vi "STM32.cmd.vi"(8 "Error In":errorcluster caption="错误输入", 10 "命令":string, 11 "VISA资源输入":refnum<visa-resource-name>) -> (0 "Error Out":errorcluster caption="错误输出", 1 "附加数据":string, 2 "返回":string, 3 "返回长度":u32)   [LabVIEW 2012, in "Lib_UEL.ATE.lvlib" / "STM32-CoreBD.lvlib"]
uses:
  STM32-CoreBD.lvlib
  <vilib>/Instr/_visa.llb/VISA Open Access Mode.ctl
panel:
  out "返回数":u32
  out "附加读取长度":u32
  out "读取缓冲区":string
  out "发送长度":u32
  out "错误码解析":T1(ring)
  out "数据长度":u8
  # "Version History\nV01,2014-4-14, 初始版本."
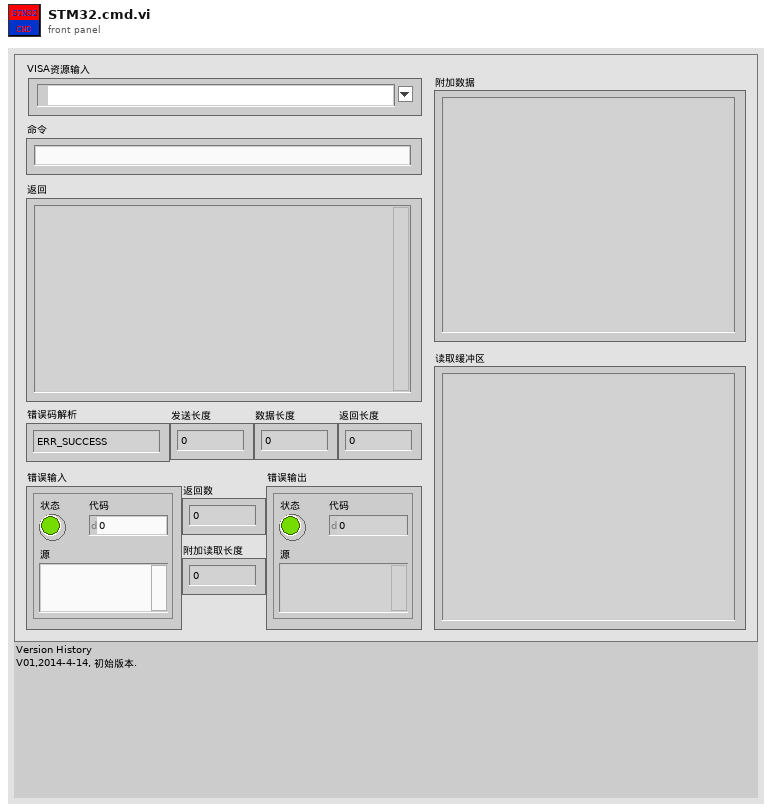
[diagram p1: front panel]
types:
  T1 = enum16{"ERR_SUCCESS", "ERR_SYSTEM", "ERR_POWER", "ERR_SYS_RESERVE\t", "ERR_SYS_RESERVE1", "ERR_SYS_RESERVE2", "ERR_SYS_RESERVE3", "ERR_SYS_RESERVE4", "ERR_SYS_UNDEFINED\t", "ERR_ADC_RESERVE", "ERR_ADC_RESERVE1", "ERR_ADC_RESERVE2", "ERR_ADC_RESERVE3", "ERR_ADC_INIT\t", "ERR_ADC_PARA", "ERR_ADC_USED\t", "ERR_ADC_UNDEFINED\t", "ERR_DAC_RESERVE\t", "ERR_DAC_RESERVE1\t", "ERR_DAC_RESERVE2\t", "ERR_DAC_RESERVE3", "ERR_DAC_INIT", "ERR_DAC_PARA", "ERR_DAC_USED", "ERR_DAC_UNDEFINED", "ERR_SDIO_COMM\t", "ERR_SDIO_RESERVE\t", "ERR_SDIO_RESERVE1", "ERR_SDIO_RESERVE2", "ERR_SDIO_NONECARD", "ERR_SDIO_INIT\t", "ERR_SDIO_RECONNECT", "ERR_SDIO_UNDEFINED", "ERR_USB_RESERVE", "ERR_USB_RESERVE1", "ERR_USB_RESERVE2", "ERR_USB_RESERVE3\t", "ERR_USB_RESERVE4", "ERR_USB_RESERVE5\t", "ERR_USB_RESERVE6\t", "ERR_USB_UNDEFINED\t", "ERR_FS_RESERVE\t", "ERR_FS_RESERVE1\t", "ERR_FS_RESERVE2", "ERR_FS_RESERVE3\t", "ERR_FS_INIT\t", "ERR_FS_NOFILE", "ERR_FS_OFFLINE\t", "ERR_FS_UNDEFINED", "1", "2", "3", "4", "5", "6", "7", "8", "9", "10", "11", "12", "13", "14", "15", "16", "17", "18", "19", "20", "21", "22", "23", "24", "25", "26", "27", "28", "29", "30", "31", "32", "33", "34", "35", "36", "37", "38", "39", "40", "41", "42", "43", "44", "45", "46", "47", "48", "49", "50", "51", "52", "53", "54", "55", "56", "57", "58", "59", "60", "61", "62", "63", "64", "65", "66", "67", "68", "69", "70", "71", "72", "73", "74", "75", "76", "77", "78", "79", "80", "81", "82", "ERR_SCPI_SPECIALREPLY", "ERR_SCPI_NOCMD", "ERR_SCPI_CMDFORMAT", "ERR_SCPI_PARAFORMAT", "ERR_SCPI_NONSUPPORT\t"}
  T2 = typedef "VISA Open Access Mode.ctl" = u32
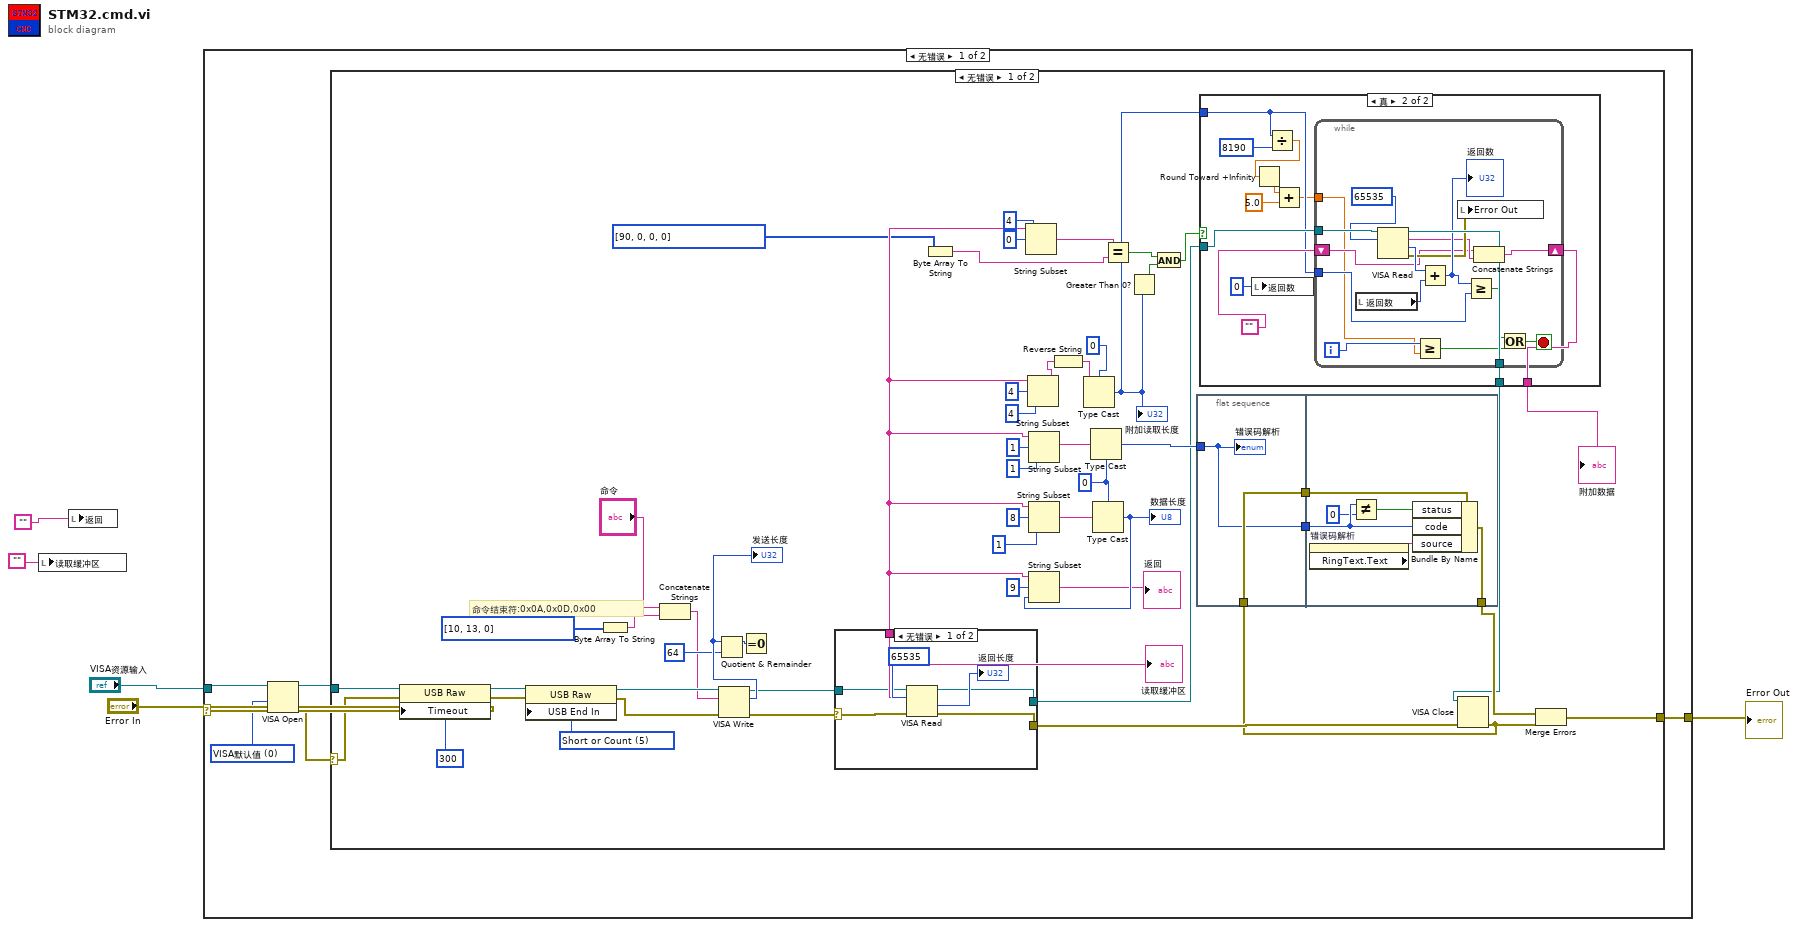
[diagram p0: block diagram]
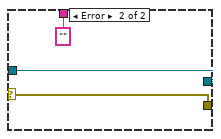
[diagram p2: hidden frame]
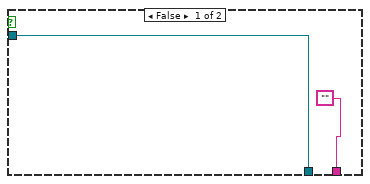
[diagram p3: hidden frame]
diagram:
  n1 = local write "读取缓冲区"("") -> ()
  n2 = local write "返回"("") -> ()
  n3 = case shown="无错误" "Error In" {
    selector: "Error In" -> [w10 w112]
    tunnel: [w6 w112] -> w1
    tunnel: "VISA资源输入" -> [w8 _]
    frame No Error {
      w11 = T2 0 items=["VISA默认值"=0, "排它锁定"=1, "加载已配置的设置"=4] ("Access Mode")
      n4 = VISA Open(access mode=w11, error in (no error)=w10, VISA resource name=w8) -> (VISA resource name=w9:refnum<visa-resource-name>, error out=w7:errorcluster)  [unwired: 2 in]
      n5 = case shown="无错误" w7 {
        selector: w7 -> [w18 w111]
        tunnel: [w47 w111] -> w6
        tunnel: w9 -> [w42 _]
        frame No Error {
          w36 = u16 5 items=["None"=0, "Short"=4, "Short or Count"=5] ("USB Settings:End Mode for Reads")
          w44 = u8 0
          # "命令结束符:0x0A,0x0D,0x00"
          n6 = property class="USB Raw"(reference=w42, error in=w18, "Timeout"=u32 300 ("General Settings:Timeout Value")) -> (reference out=w40:refnum<visa-resource-name>, error out=w39:errorcluster)
          n7 = property class="USB Raw"(reference=w40, error in=w39, "USB End In"=w36) -> (reference out=w38:refnum<visa-resource-name>, error out=w37:errorcluster)
          n8 = Byte Array To String(unsigned byte array=u8[] [10, 13, 0]) -> (string=w12:string)
          n9 = Concatenate Strings("命令", w12) -> (w14:string)
          n10 = VISA Write(VISA resource name=w38, write buffer=w14, error in (no error)=w37) -> (VISA resource name out=w17:refnum<visa-resource-name>, return count=w21:u32, error out=w16:errorcluster)
          "发送长度" <- w21
          n11 = Quotient & Remainder(x=w21, y=u32 64) -> (x-y*floor(x/y)=w19:u32)  [unwired: 1 out]
          n12 = Equal To 0?(x=w19) -> ()  [unwired: 1 out]
          n13 = case shown="无错误" w16 {
            selector: w16 -> [w64 w71]
            tunnel: [w69 w71] -> w61
            tunnel: [w67 w72] -> w43
            tunnel: [w66 "" ("read buffer")] -> w31
            tunnel: w17 -> [w65 w72]
            frame No Error {
              n14 = VISA Read(VISA resource name=w65, byte count=u32 65535 ("字节总数"), error in (no error)=w64) -> (VISA resource name out=w67:refnum<visa-resource-name>, read buffer=w66:string, return count=→"返回长度":u32, error out=w69:errorcluster)
            }
            frame Error {
            }
          }
          "读取缓冲区" <- w31
          n15 = Byte Array To String(unsigned byte array=i32[] [90, 0, 0, 0]) -> (string=w26:string)
          n16 = String Subset(string=w31, offset (0)=0 ("偏移量(0)"), length (rest)=4 ("长度（剩余）")) -> (substring=w29:string)
          n17 = String Subset(string=w31, offset (0)=4 ("偏移量(0)"), length (rest)=4 ("长度（剩余）")) -> (substring=w34:string)
          n18 = String Subset(string=w31, offset (0)=1 ("偏移量(0)"), length (rest)=1 ("长度（剩余）")) -> (substring=w53:string)
          n19 = String Subset(string=w31, offset (0)=8 ("偏移量(0)"), length (rest)=1 ("长度（剩余）")) -> (substring=w55:string)
          n20 = Reverse String(1:w34) -> (0:w33:string)
          n21 = Type Cast(type=u32 0, x=w33) -> (*(type *) &x=w32:u32)
          "附加读取长度" <- w32
          n22 = Type Cast(type=w44, x=w53) -> (*(type *) &x=w50:u8)
          n23 = Type Cast(type=w44, x=w55) -> (*(type *) &x=w54:u8)
          "数据长度" <- w54
          n24 = String Subset(string=w31, offset (0)=9 ("偏移量(0)"), length (rest)=w54) -> (substring=→"返回":string)
          n25 = Equal?(x=w29, y=w26) -> (x = y?=w24:bool)
          n26 = Greater Than 0?(x=w32) -> (x > 0?=w25:bool)
          n27 = And(x=w24, y=w25) -> (x .and. y?=w23:bool)
          n28 = flat-sequence {
            tunnel: w50 -> [w103]
            tunnel: [w104] -> w63
            tunnel: w49 -> [w104]
            tunnel: [w103] -> w62
            tunnel: w63 -> [w109]
            tunnel: w62 -> [w108]
            tunnel: [w105] -> w48
            frame #0 {
              "错误码解析" <- w103
            }
            frame #1 {
              n29 = property on="错误码解析" class="Enum (严格)"() -> ("RingText.Text"=w110:string)  [unwired: 2 in, 2 out]
              n30 = Not Equal?(x=w108, y=u8 0) -> (x != y?=w106:bool)
              n31 = Bundle By Name(cluster=w109, "status"=w106, "code"=w108, "source"=w110) -> (w105:errorcluster)
            }
          }
          n32 = case shown="真" w23 {
            tunnel: w32 -> [_ w77]
            tunnel: w43 -> [w75 w86]
            tunnel: [w75 w85] -> w22
            tunnel: ["" w82] -> w15
            frame False {
            }
            frame True {
              n33 = local write "返回数"(u32 0 ("返回数")) -> ()
              n34 = Divide(x=w77, y=u32 8190 ("字节总数")) -> (x/y=w80:dbl)
              n35 = Round Toward +Infinity(x=w80) -> (ceil(x): smallest int >= x=w79:dbl)
              n36 = Add(x=w79, y=5.0) -> (x+y=w76:dbl)
              n37 = while {
                tunnel: w86 -> [w102]
                tunnel: [w101] -> w85
                tunnel: w77 -> [w97]
                shift-right: [w93] -> w82
                shift-left: "" -> [w94]
                tunnel: w76 -> [w89]
                i -> [w90]
                stop <- w92 stop-if-true
                n38 = local read "返回数"() -> (w99:u32)
                n39 = VISA Read(VISA resource name=w102, byte count=u32 65535 ("字节总数")) -> (VISA resource name out=w101:refnum<visa-resource-name>, read buffer=w95:string, return count=w100:u32, error out=w96:errorcluster)  [unwired: 1 in]
                n40 = Greater Or Equal?(x=w90, y=w89) -> (x >= y?=w88:bool)
                n41 = Add(x=w100, y=w99) -> (x+y=w98:u32)
                "返回数" <- w98
                n42 = local write "Error Out"(w96) -> ()
                n43 = Greater Or Equal?(x=w98, y=w97) -> (x >= y?=w91:bool)
                n44 = Concatenate Strings(w94, w95) -> (w93:string)
                n45 = Or(x=w91, y=w88) -> (x .or. y?=w92:bool)
              }
            }
          }
          "附加数据" <- w15
          n46 = VISA Close(VISA resource name=w22, error in (no error)=w61) -> (error out=w49:errorcluster)
          n47 = Merge Errors(w48, w49) -> (w47:errorcluster)
        }
        frame Error {
        }
      }
    }
    frame Error {
    }
  }
  "Error Out" <- w1
